vi "sub_joystick_master.vi"(8 "error in":errorcluster) -> (0 "error out":errorcluster)   [LabVIEW 2019]
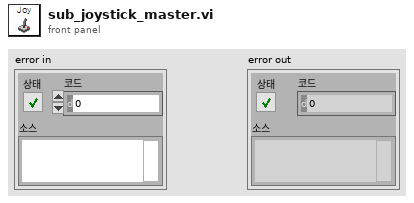
[diagram p1: front panel]
types:
  T1 = enum16{"enable", "init", "read", "write joystick", "write manual"}
  T2 = cluster{"axis info":cluster{"X axis":i32, "Y axis":i32, "Z axis":i32, "X axis rotation":i32, "Y axis rotation":i32, "Z axis rotation":i32, "U axis":i32, "V axis":i32}, "button info":cluster{"button 1":bool, "button 2":bool, "button 3":bool, "button 4":bool, "button 5":bool, "button 6":bool, "button 7":bool, "button 8":bool, "button 9":bool, "button 10":bool, "button 11":bool, "button 12":bool, "button 13":bool, "button 14":bool, "button 15":bool, "button 16":bool, "button 17":bool, "button 18":bool, "button 19":bool, "button 20":bool, "button 21":bool, "button 22":bool, "button 23":bool, "button 24":bool, "button 25":bool, "button 26":bool, "button 27":bool, "button 28":bool, "button 29":bool, "button 30":bool, "button 31":bool, "button 32":bool}, "direction info":cluster{"pov 1":i32, "pov 2":i32, "pov 3":i32, "pov 4":i32}}
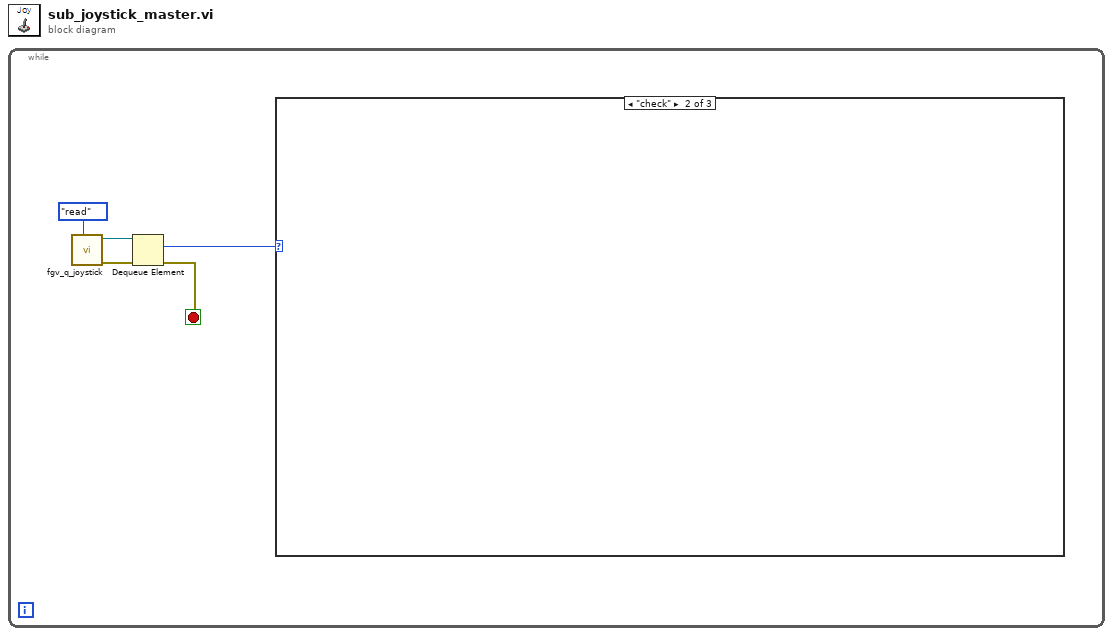
[diagram p0: block diagram]
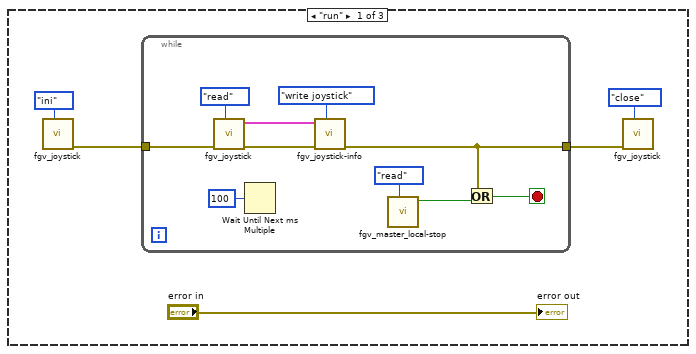
[diagram p2: hidden frame]
diagram:
  n1 = while {
    stop <- w1 stop-if-true
    n2 = call "fgv_q_joystick.vi"("cmd"=enum16{"create", "write", "read", "close"}."read") -> ("error out"=w4:errorcluster, "queue out"=w3:refnum<queue>)  [unwired: 9 in]
    n3 = Dequeue Element(queue=w3, error in (no error)=w4) -> (element=w2:enum16{"run", "check", "stop"}, error out=w1:errorcluster)  [unwired: 1 in, 2 out]
    n4 = case shown="\"check\"" w2 {
      frame "run" {
        n5 = call "fgv_joystick.vi"("cmd"=enum16{"ini", "read", "close"}."ini") -> ("error out"=w9:errorcluster)  [unwired: 9 in, 1 out]
        n6 = while {
          tunnel: w9 -> [w18]
          tunnel: [w16] -> w10
          stop <- w19 stop-if-true
          n7 = call "fgv_joystick.vi"("cmd"=enum16{"ini", "read", "close"}."read", "error in"=w18) -> ("error out"=w17:errorcluster, "joystick info-out"=w14:T2)  [unwired: 8 in]
          n8 = Wait Until Next ms Multiple(millisecond multiple=u32 100 ("milliseconds to wait")) -> ()  [unwired: 1 out]
          n9 = call "fgv_joystick-info.vi"("init"=T1."write joystick", "error in"=w17, "joystick info-in"=w14) -> ("error out"=w16:errorcluster)  [unwired: 5 in, 3 out]
          n10 = call "fgv_master_local-stop.vi"("cmd"=enum16{"init", "read", "stop"}."read") -> ("out"=w11:bool)  [unwired: 10 in]
          n11 = Or(x=w16, y=w11) -> (x .or. y?=w19:bool)
        }
        n12 = call "fgv_joystick.vi"("cmd"=enum16{"ini", "read", "close"}."close", "error in"=w10) -> ()  [unwired: 8 in, 2 out]
        "error out" <- "error in"
      }
      frame "check" {
      }
      frame "stop", Default {
      }
    }
  }
